vi "FileOptimize.vi"(8 "error in (no error)":errorcluster, 11 "controller in":refnum<k24>) -> (0 "error out":errorcluster, 3 "controller out":refnum<k24>)   [LabVIEW 2010]
uses:
  c:/aerotech/controller/5.xx.xxx/ensemble/pc/labview/2010/bin/Aerotech.Ensemble.dll
  bin/Aerotech.Ensemble.dll
  c:/aerotech/controller/5.xx.xxx/ensemble/pc/labview/2010/bin/Aerotech.Ensemble.LabVIEW.dll
  bin/Aerotech.Ensemble.LabVIEW.dll
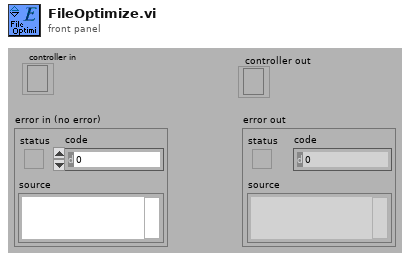
[diagram p1: front panel]
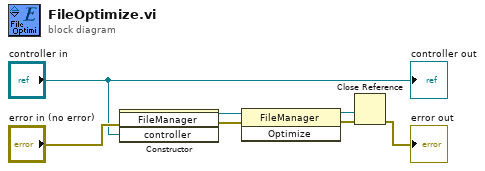
[diagram p0: block diagram]
diagram:
  n1 = constructor class="FileManager"(error in="error in (no error)", "controller"="controller in") -> (reference out=w1:refnum<k24>, error out=w3:errorcluster)  [unwired: 2 in, 2 out]
  n2 = invoke class="FileManager" method="Optimize"(reference=w1, error in=w3) -> (reference out=w6:refnum<k24>, error out=w7:errorcluster)  [unwired: 1 in, 1 out]
  n3 = Close Reference(reference=w6, error in (no error)=w7) -> (error out=→"error out":errorcluster)
  "controller out" <- "controller in"
